vi "Post-Build Action.vi"(5 "Files Generated by Build":path[](array[path]), 6 "Top Level/Always Included VIs":path[](array[path]), 7 "Destination Path":path, 8 "error in (no error)":errorcluster, 9 "Target Name":string, 10 "Build Specification Name":string, 11 "Project Path":path) -> (0 "error out":errorcluster)   [LabVIEW 2013]
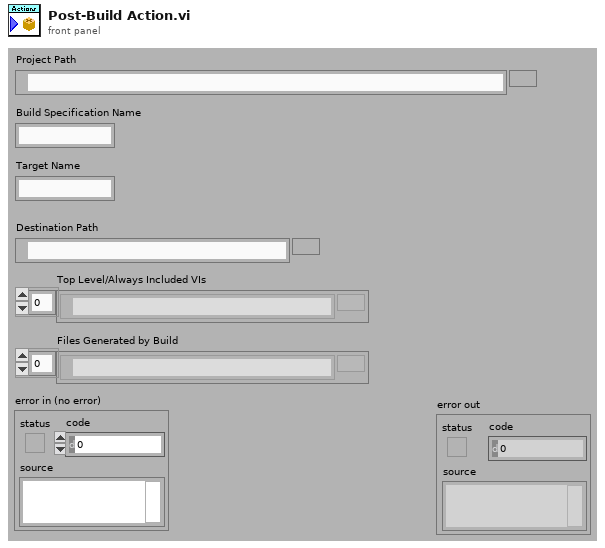
[diagram p1: front panel]
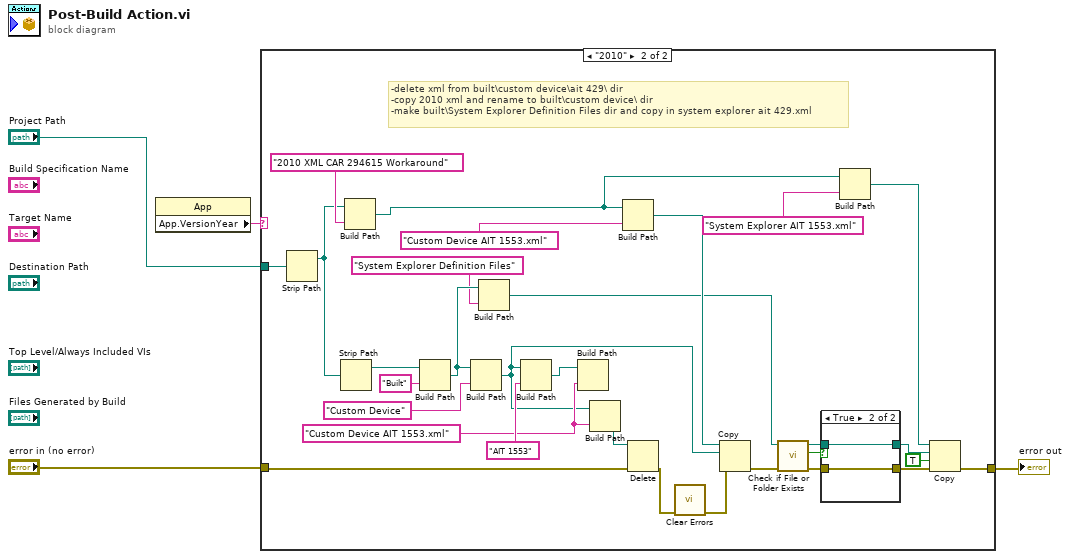
[diagram p0: block diagram]
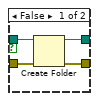
[diagram p3: hidden frame]
diagram:
  n1 = property class="App"() -> ("App.VersionYear"=w4:string)  [unwired: 2 in, 2 out]
  n2 = case shown="\"2010\"" w4 {
    tunnel: "error in (no error)" -> [w5 w33]
    tunnel: "Project Path" -> [_ w13]
    tunnel: [w5 w17] -> w1
    frame Default {
    }
    frame "2010" {
      w10 = "Custom Device AIT 1553.xml" ("name or relative path")
      # "-delete xml from built\\custom device\\ait 429\\ dir\n-copy 2010 xml and rename to built\\custom device\\ dir\n-make built\\System Explorer Definition Files dir and copy in system explorer ait 429.xml"
      n3 = Strip Path(path=w13) -> (stripped path=w7:path)  [unwired: 1 out]
      n4 = Strip Path(path=w7) -> (stripped path=w12:path)  [unwired: 1 out]
      n5 = Build Path(base path=w7, name or relative path="2010 XML CAR 294615 Workaround") -> (appended path=w22:path)
      n6 = Build Path(base path=w12, name or relative path="Built") -> (appended path=w28:path)
      n7 = Build Path(base path=w28, name or relative path="Custom Device") -> (appended path=w9:path)
      n8 = Build Path(base path=w28, name or relative path="System Explorer Definition Files") -> (appended path=w26:path)
      n9 = Build Path(base path=w9, name or relative path="AIT 1553") -> (appended path=w11:path)
      n10 = Build Path(base path=w11, name or relative path=w10) -> ()  [unwired: 1 out]
      n11 = Build Path(base path=w9, name or relative path=w10) -> (appended path=w8:path)
      n12 = Build Path(base path=w22, name or relative path="Custom Device AIT 1553.xml") -> (appended path=w30:path)
      n13 = Delete(path (use dialog)=w8, error in=w33) -> (error out=w15:errorcluster)  [unwired: 3 in, 2 out]
      n14 = call <vilib>:"Clear Errors.vi"("error in (no error)"=w15) -> ("error out"=w14:errorcluster)  [unwired: 6 in]
      n15 = Copy(8:w14, 10:w9, 11:w30) -> (0:w29:errorcluster)  [unwired: 2 in, 2 out]
      n16 = call <vilib>:"Check if File or Folder Exists.vi"("error in (no error)"=w29, "path"=w26) -> ("error out"=w24:errorcluster, "file or folder exists?"=w25:bool, "dup path"=w23:path)  [unwired: 7 in]
      n17 = case shown="True" w25 {
        tunnel: w24 -> [w39 w41]
        tunnel: w23 -> [w38 w40]
        tunnel: [w37 w41] -> w20
        tunnel: [w36 w40] -> w19
        frame False {
          n18 = Create Folder(path (use dialog)=w38, error in=w39) -> (created path=w36:path, error out=w37:errorcluster)  [unwired: 1 in, 1 out]
        }
        frame True {
        }
      }
      n19 = Build Path(base path=w22, name or relative path="System Explorer AIT 1553.xml") -> (appended path=w18:path)
      n20 = Copy(8:w20, 9:TRUE ("overwrite (F)"), 10:w19, 11:w18) -> (0:w17:errorcluster)  [unwired: 1 in, 2 out]
    }
  }
  "error out" <- w1
